vi "Trigger Conditions Check.vi"(7 "Force Trigger?":bool, 8 "error in (no error)":errorcluster, 9 "Waveform Data":waveform(dbl)[](array[waveform]), 11 "Acq and Logging Props":T1) -> (0 "error out":errorcluster, 3 "Trigger Condition Met?":bool)   [LabVIEW 2013]
uses:
  <vilib>/Analysis/5stat.llb/RMS (DBL).vi
  <vilib>/Analysis/NI_AALPro.lvlib
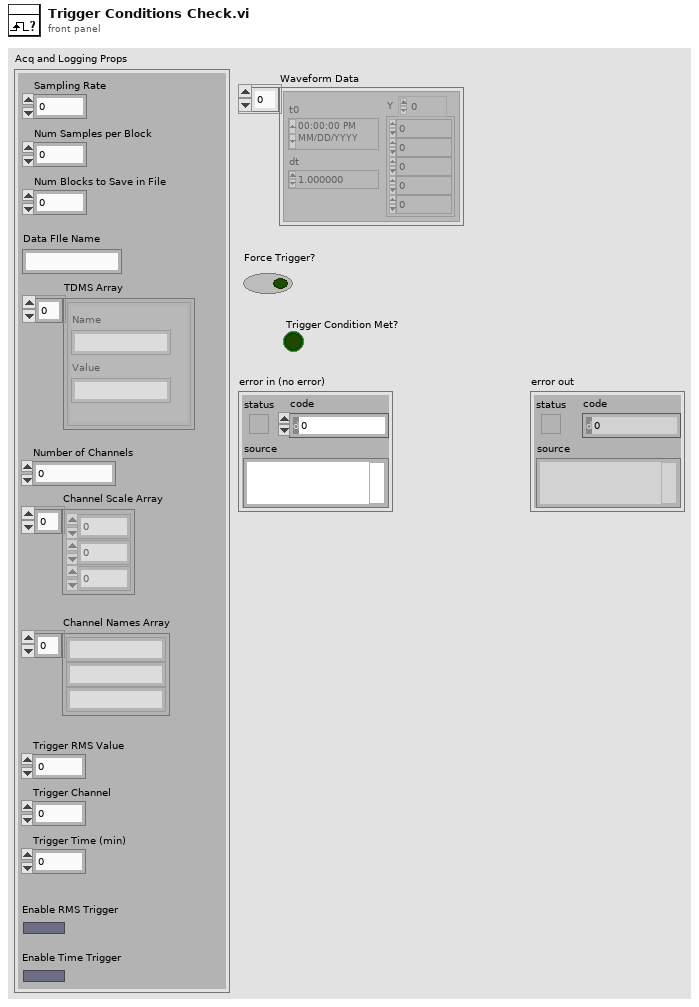
[diagram p1: front panel]
types:
  T1 = cluster{"Sampling Rate":dbl, "Num Samples per Block":i32, "Num Blocks to Save in File":i32, "Data FIle Name":string, "TDMS Array":cluster{"Name":string, "Value":string}[], "Number of Channels":i32, "Channel Scale Array":dbl[], "Channel Names Array":string[], "Trigger RMS Value":dbl, "Trigger Channel":i32, "Trigger Time (min)":i32, "Enable RMS Trigger":bool, "Enable Time Trigger":bool}
  T2 = typedef "LVDateTimeRec.ctl" = cluster{"fractional second":dbl, "second":i32, "minute":i32, "hour":i32, "day of month":i32, "month":i32, "year":i32, "day of week":i32, "day of year":i32, "DST":i32}
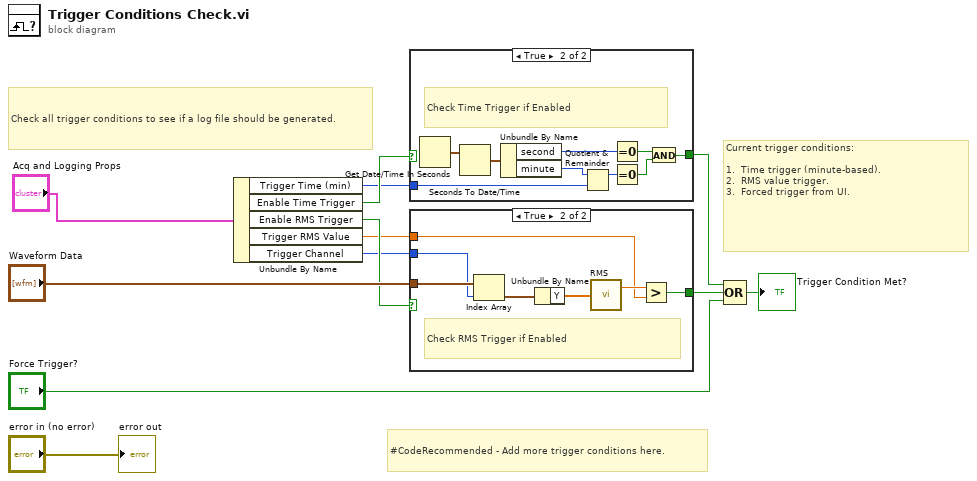
[diagram p0: block diagram]
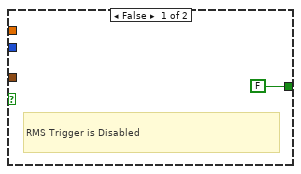
[diagram p2: hidden frame]
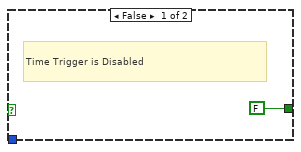
[diagram p3: hidden frame]
diagram:
  # "Check all trigger conditions to see if a log file should be generated."
  # "Current trigger conditions:\n\n1.  Time trigger (minute-based).\n2.  RMS value trigger.\n3.  Forced trigger from UI."
  # "#CodeRecommended - Add more trigger conditions here."
  n1 = Unbundle By Name("Acq and Logging Props") -> ("Trigger Time (min)"=w4:i32, "Enable Time Trigger"=w8:bool, "Enable RMS Trigger"=w7:bool, "Trigger RMS Value"=w2:dbl, "Trigger Channel"=w3:i32)
  n2 = case shown="True" w8 {
    tunnel: [FALSE w15] -> w5
    tunnel: w4 -> [_ w14]
    frame False {
      # "Time Trigger is Disabled"
    }
    frame True {
      # "Check Time Trigger if Enabled"
      n3 = Get Date/Time In Seconds() -> (seconds since 1Jan1904=w19:timestamp)
      n4 = Seconds To Date/Time(time stamp (now)=w19) -> (date time rec=w22:T2)  [unwired: 1 out]
      n5 = Unbundle By Name(w22) -> ("second"=w21:i32, "minute"=w18:i32)
      n6 = Quotient & Remainder(x=w18, y=w14) -> (x-y*floor(x/y)=w17:i32)  [unwired: 1 out]
      n7 = Equal To 0?(x=w21) -> (x = 0?=w20:bool)
      n8 = Equal To 0?(x=w17) -> (x = 0?=w16:bool)
      n9 = And(x=w20, y=w16) -> (x .and. y?=w15:bool)
    }
  }
  n10 = case shown="True" w7 {
    tunnel: "Waveform Data" -> [_ w30]
    tunnel: [FALSE w29] -> w10
    tunnel: w3 -> [_ w25]
    tunnel: w2 -> [_ w24]
    frame False {
      # "RMS Trigger is Disabled"
    }
    frame True {
      # "Check RMS Trigger if Enabled"
      n11 = Index Array(array=w30, index=w25) -> (element=w26:waveform(dbl))
      n12 = Unbundle By Name(w26) -> ("Y"=w28:dbl[])
      n13 = call-poly <vilib>:"RMS.vi"("X"=w28) -> ("rms value"=w27:dbl)  [unwired: 1 out]
      n14 = Greater?(x=w27, y=w24) -> (0:w29:bool)
    }
  }
  n15 = Compound Arithmetic op=OR(w5, w10, "Force Trigger?") -> (→"Trigger Condition Met?":bool)
  "error out" <- "error in (no error)"
